vi "Auto Ball Pickup.vi"(8 "error in":errorcluster) -> ()   [LabVIEW 2013]
uses:
  Auto Ball States.ctl
  Intake Actions.ctl
  Auto Pickup Global.vi
panel:
  in  "Hysterisis":dbl=4.0
  in  "Far Distance":dbl=30.0
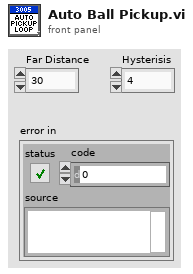
[diagram p1: front panel]
types:
  T1 = typedef "Auto Ball States.ctl" = enum16{"Off", "Start", "Idle", "Found", "Lost", "Contained"}
  T2 = typedef "WPI_DigitalInputDevRef.ctl" = cluster{"DevStatus":errorcluster, "DIO Channel":T3, "Digital Module":T4}
  T3 = typedef "FPGA_DIOChannel.ctl" = enum8{"DIO 1", "DIO 2", "DIO 3", "DIO 4", "DIO 5", "DIO 6", "DIO 7", "DIO 8", "DIO 9", "DIO 10", "DIO 11", "DIO 12", "DIO 13", "DIO 14", "Invalid"}
  T4 = typedef "FPGA_TypedefDigitalModule.ctl" = enum16{"Digital Module 1", "Digital Module 2"}
  T5 = typedef "WPI_CounterDevRef.ctl" = cluster{"DevStatus":errorcluster, "CntIndex":T6}
  T6 = typedef "FPGA_CounterCtrSystemIndex.ctl" = enum8{"Ctr 0", "Ctr 1", "Ctr 2", "Ctr 3", "Ctr 4", "Ctr 5", "Ctr 6", "Ctr 7", "Invalid"}
  T7 = typedef "Intake Actions.ctl" = enum16{"Extend", "Contain", "Motor Still", "Motor Outward", "Motor Inward", "Collect", "Pass", "Herd", "Contain Off", "Collect Delay Off", "Patea"}
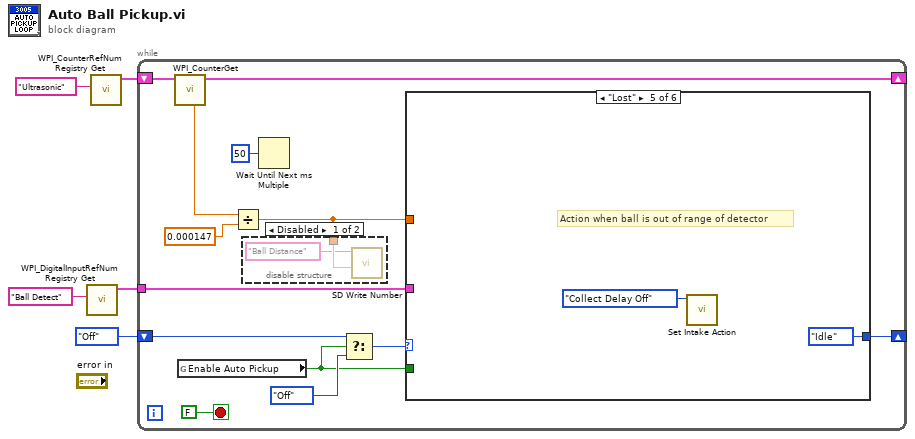
[diagram p0: block diagram]
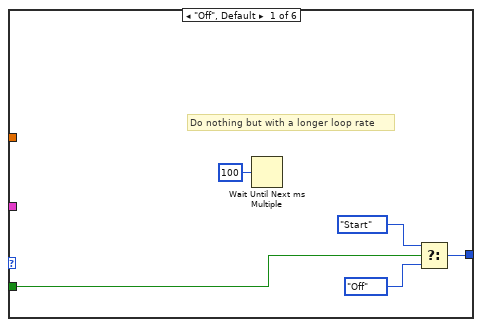
[diagram p3: hidden frame]
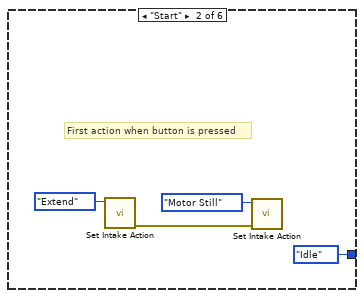
[diagram p4: hidden frame]
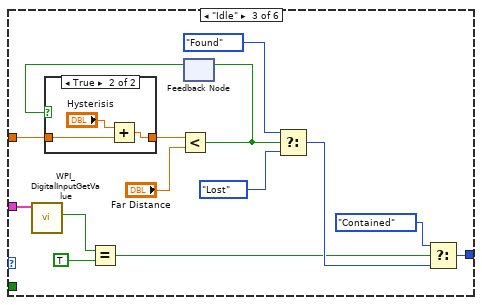
[diagram p5: hidden frame]
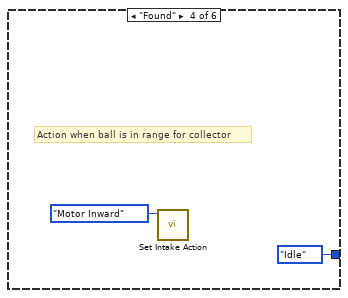
[diagram p7: hidden frame]
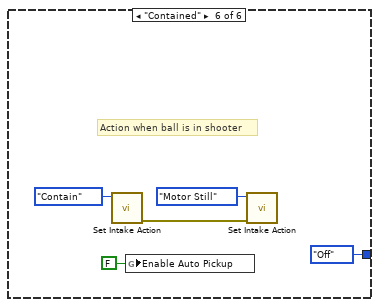
[diagram p8: hidden frame]
diagram:
  n1 = call <vilib>:"WPI_DigitalInputRefNum Registry Get.vi"("refnum name"="Ball Detect") -> ("DigitalInputDevRef"=w1:T2)  [unwired: 9 in, 1 out]
  n2 = call <vilib>:"WPI_CounterRefNum Registry Get.vi"("refnum name"="Ultrasonic") -> ("CounterDevRef"=w4:T5)  [unwired: 9 in, 1 out]
  n3 = while {
    shift-right: [w10] -> _
    shift-left: Auto_Ball_States."Off" -> [w17]
    shift-right: [w12] -> _
    shift-left: w4 -> [w13]
    tunnel: w1 -> [w6]
    stop <- FALSE stop-if-true
    n4 = call <vilib>:"WPI_CounterGet.vi"("CounterDevRef in"=w13) -> ("CounterDevRef out"=w12:T5, "Period (sec)"=w14:dbl)  [unwired: 5 in, 4 out]
    n5 = global read "Auto Pickup Global.vi" "Enable Auto Pickup"() -> (w7:bool)
    n6 = Divide(x=w14, y=0.000147 ("Scaling factor (s/in)")) -> (x/y=w9:dbl)
    n7 = disable-structure shown="Disabled" {
      disable-tunnel: w9 -> [w20 _]
      frame Disabled {
        n8 = call <vilib>:"SD Write Number.vi"("Numeric"=w20, "Name"="Ball Distance") -> ()  [unwired: 8 in, 2 out]
      }
      frame Enabled {
      }
    }
    n9 = Wait Until Next ms Multiple(millisecond multiple=u32 50) -> ()  [unwired: 1 out]
    n10 = Select(t=w17, s=w7, f=Auto_Ball_States."Off") -> (s? t:f=w16:T1)
    n11 = case shown="\"Lost\"" w16 {
      tunnel: w9 -> [_ _ w32 _ _ _]
      tunnel: [w25 Auto_Ball_States."Idle" w41 Auto_Ball_States."Idle" Auto_Ball_States."Idle" Auto_Ball_States."Off"] -> w10
      tunnel: w7 -> [w22 _ _ _ _ _]
      tunnel: w6 -> [_ _ w35 _ _ _]
      frame "Off", Default {
        # "Do nothing but with a longer loop rate"
        n12 = Wait Until Next ms Multiple(millisecond multiple=u32 100) -> ()  [unwired: 1 out]
        n13 = Select(t=Auto_Ball_States."Start", s=w22, f=Auto_Ball_States."Off") -> (s? t:f=w25:T1)
      }
      frame "Start" {
        # "First action when button is pressed"
        n14 = call "Set Intake Action.vi"("Action"=Intake_Actions."Extend") -> ("error out"=w27:errorcluster)  [unwired: 10 in]
        n15 = call "Set Intake Action.vi"("error in"=w27, "Action"=Intake_Actions."Motor Still") -> ()  [unwired: 9 in, 1 out]
      }
      frame "Idle" {
        n16 = call <vilib>:"WPI_DigitalInputGetValue.vi"("DigitalInputDevRef"=w35) -> ("Value"=w36:bool)  [unwired: 8 in, 2 out]
        n17 = Equal?(x=w36, y=TRUE ("x")) -> (x = y?=w34:bool)
        n18 = feedback #1() -> (w30:bool)  [unwired: 1 in]
        n19 = case shown="True" w30 {
          tunnel: w32 -> [w44 w46]
          tunnel: [w44 w45] -> w31
          frame False {
          }
          frame True {
            n20 = Add(x="Hysterisis", y=w46) -> (x+y=w45:dbl)
          }
        }
        n21 = Less?(x=w31, y="Far Distance") -> (x < y?=w33:bool)
        n22 = feedback-in #1(w33) -> ()
        n23 = Select(t=Auto_Ball_States."Found", s=w33, f=Auto_Ball_States."Lost") -> (s? t:f=w42:T1)
        n24 = Select(t=Auto_Ball_States."Contained", s=w34, f=w42) -> (s? t:f=w41:T1)
      }
      frame "Found" {
        # "Action when ball is in range for collector"
        n25 = call "Set Intake Action.vi"("Action"=Intake_Actions."Motor Inward") -> ()  [unwired: 10 in, 1 out]
      }
      frame "Lost" {
        # "Action when ball is out of range of detector"
        n26 = call "Set Intake Action.vi"("Action"=Intake_Actions."Collect Delay Off") -> ()  [unwired: 10 in, 1 out]
      }
      frame "Contained" {
        # "Action when ball is in shooter"
        n27 = call "Set Intake Action.vi"("Action"=Intake_Actions."Contain") -> ("error out"=w53:errorcluster)  [unwired: 10 in]
        n28 = global write "Auto Pickup Global.vi" "Enable Auto Pickup"(FALSE ("Enable Auto Pickup")) -> ()
        n29 = call "Set Intake Action.vi"("error in"=w53, "Action"=Intake_Actions."Motor Still") -> ()  [unwired: 9 in, 1 out]
      }
    }
  }
